vi "PrimaryInterfaceGetData.vi"(8 "PrimaryInterface":refnum<k24>, 11 "error in":errorcluster) -> (0 "Data":T1, 3 "error out":errorcluster)   [LabVIEW 2011, in "UnderAutomation.UniversalRobots.lvlib"]
uses:
  UnderAutomation.UniversalRobots.lvlib
  C:/Users/fg/Documents/UniversalRobots.vi/LabVIEW_2024/UnderAutomation.UniversalRobots/lib/UnderAutomation.UniversalRobots.dll
  LabVIEW_2024/UnderAutomation.UniversalRobots/lib/UnderAutomation.UniversalRobots.dll
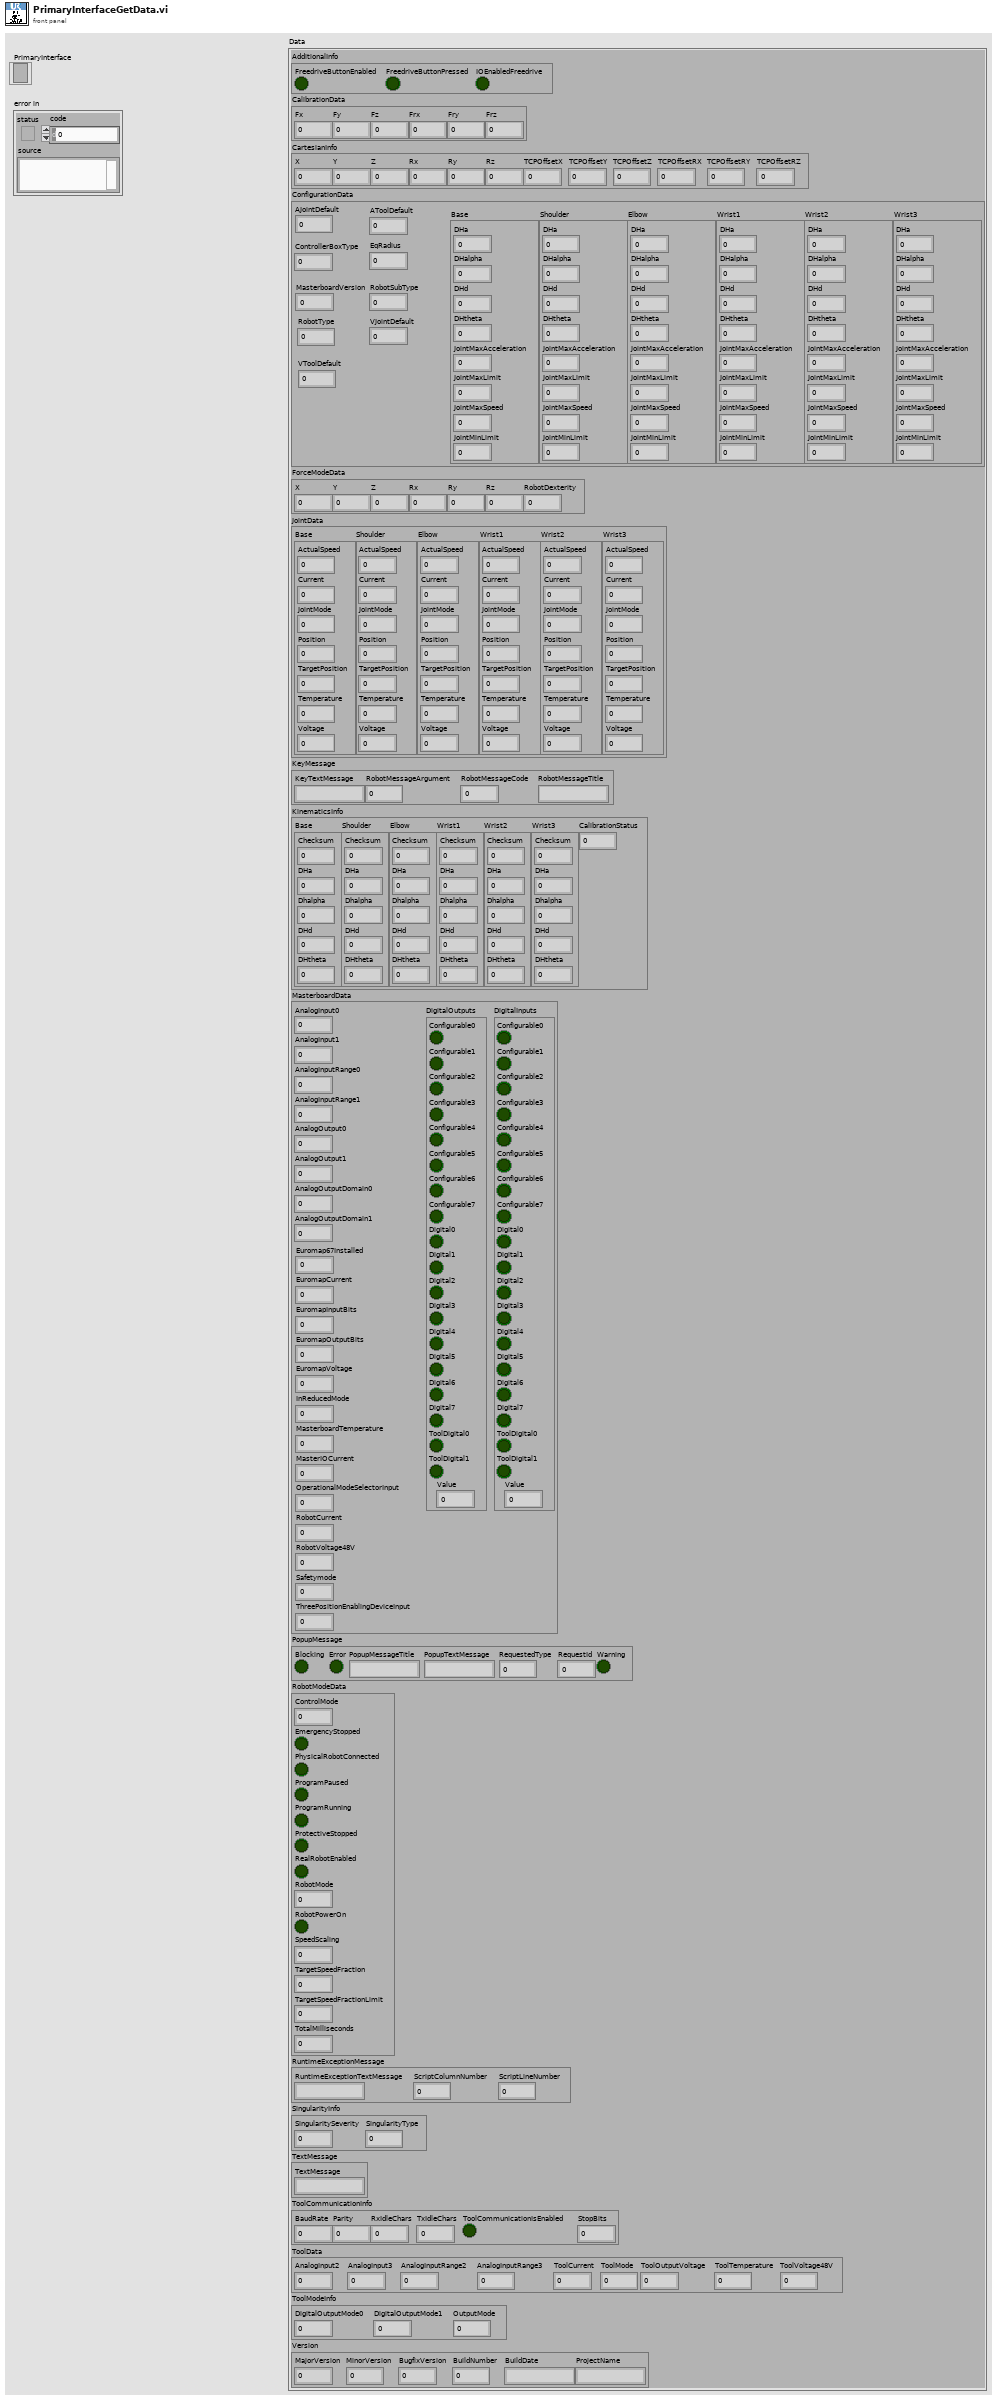
[diagram p1: front panel]
types:
  T1 = cluster{"AdditionalInfo":cluster{"FreedriveButtonEnabled":bool, "FreedriveButtonPressed":bool, "IOEnabledFreedrive":bool}, "CalibrationData":cluster{"Fx":dbl, "Fy":dbl, "Fz":dbl, "Frx":dbl, "Fry":dbl, "Frz":dbl}, "CartesianInfo":cluster{"X":dbl, "Y":dbl, "Z":dbl, "Rx":dbl, "Ry":dbl, "Rz":dbl, "TCPOffsetX":dbl, "TCPOffsetY":dbl, "TCPOffsetZ":dbl, "TCPOffsetRX":dbl, "TCPOffsetRY":dbl, "TCPOffsetRZ":dbl}, "ConfigurationData":cluster{"AJointDefault":dbl, "AToolDefault":dbl, "ControllerBoxType":i32, "EqRadius":dbl, "MasterboardVersion":i32, "RobotSubType":i32, "RobotType":i32, "VJointDefault":dbl, "VToolDefault":dbl, "Base":cluster{"DHa":dbl, "DHalpha":dbl, "DHd":dbl, "DHtheta":dbl, "JointMaxAcceleration":dbl, "JointMaxLimit":dbl, "JointMaxSpeed":dbl, "JointMinLimit":dbl}, "Shoulder":cluster{"DHa":dbl, "DHalpha":dbl, "DHd":dbl, "DHtheta":dbl, "JointMaxAcceleration":dbl, "JointMaxLimit":dbl, "JointMaxSpeed":dbl, "JointMinLimit":dbl}, "Elbow":cluster{"DHa":dbl, "DHalpha":dbl, "DHd":dbl, "DHtheta":dbl, "JointMaxAcceleration":dbl, "JointMaxLimit":dbl, "JointMaxSpeed":dbl, "JointMinLimit":dbl}, "Wrist1":cluster{"DHa":dbl, "DHalpha":dbl, "DHd":dbl, "DHtheta":dbl, "JointMaxAcceleration":dbl, "JointMaxLimit":dbl, "JointMaxSpeed":dbl, "JointMinLimit":dbl}, "Wrist2":cluster{"DHa":dbl, "DHalpha":dbl, "DHd":dbl, "DHtheta":dbl, "JointMaxAcceleration":dbl, "JointMaxLimit":dbl, "JointMaxSpeed":dbl, "JointMinLimit":dbl}, "Wrist3":cluster{"DHa":dbl, "DHalpha":dbl, "DHd":dbl, "DHtheta":dbl, "JointMaxAcceleration":dbl, "JointMaxLimit":dbl, "JointMaxSpeed":dbl, "JointMinLimit":dbl}}, "ForceModeData":cluster{"X":dbl, "Y":dbl, "Z":dbl, "Rx":dbl, "Ry":dbl, "Rz":dbl, "RobotDexterity":dbl}, "JointData":cluster{"Base":cluster{"ActualSpeed":dbl, "Current":sgl, "JointMode":u8, "Position":dbl, "TargetPosition":dbl, "Temperature":sgl, "Voltage":sgl}, "Shoulder":cluster{"ActualSpeed":dbl, "Current":sgl, "JointMode":u8, "Position":dbl, "TargetPosition":dbl, "Temperature":sgl, "Voltage":sgl}, "Elbow":cluster{"ActualSpeed":dbl, "Current":sgl, "JointMode":u8, "Position":dbl, "TargetPosition":dbl, "Temperature":sgl, "Voltage":sgl}, "Wrist1":cluster{"ActualSpeed":dbl, "Current":sgl, "JointMode":u8, "Position":dbl, "TargetPosition":dbl, "Temperature":sgl, "Voltage":sgl}, "Wrist2":cluster{"ActualSpeed":dbl, "Current":sgl, "JointMode":u8, "Position":dbl, "TargetPosition":dbl, "Temperature":sgl, "Voltage":sgl}, "Wrist3":cluster{"ActualSpeed":dbl, "Current":sgl, "JointMode":u8, "Position":dbl, "TargetPosition":dbl, "Temperature":sgl, "Voltage":sgl}}, "KeyMessage":cluster{"KeyTextMessage":string, "RobotMessageArgument":i32, "RobotMessageCode":i32, "RobotMessageTitle":string}, "KinematicsInfo":cluster{"Base":cluster{"Checksum":i32, "DHa":dbl, "Dhalpha":dbl, "DHd":dbl, "DHtheta":dbl}, "Shoulder":cluster{"Checksum":i32, "DHa":dbl, "Dhalpha":dbl, "DHd":dbl, "DHtheta":dbl}, "Elbow":cluster{"Checksum":i32, "DHa":dbl, "Dhalpha":dbl, "DHd":dbl, "DHtheta":dbl}, "Wrist1":cluster{"Checksum":i32, "DHa":dbl, "Dhalpha":dbl, "DHd":dbl, "DHtheta":dbl}, "Wrist2":cluster{"Checksum":i32, "DHa":dbl, "Dhalpha":dbl, "DHd":dbl, "DHtheta":dbl}, "Wrist3":cluster{"Checksum":i32, "DHa":dbl, "Dhalpha":dbl, "DHd":dbl, "DHtheta":dbl}, "CalibrationStatus":i32}, "MasterboardData":cluster{"AnalogInput0":dbl, "AnalogInput1":dbl, "AnalogInputRange0":i32, "AnalogInputRange1":i32, "AnalogOutput0":dbl, "AnalogOutput1":dbl, "AnalogOutputDomain0":i32, "AnalogOutputDomain1":i32, "DigitalInputs":cluster{"Configurable0":bool, "Configurable1":bool, "Configurable2":bool, "Configurable3":bool, "Configurable4":bool, "Configurable5":bool, "Configurable6":bool, "Configurable7":bool, "Digital0":bool, "Digital1":bool, "Digital2":bool, "Digital3":bool, "Digital4":bool, "Digital5":bool, "Digital6":bool, "Digital7":bool, "ToolDigital0":bool, "ToolDigital1":bool, "Value":i32}, "DigitalOutputs":cluster{"Configurable0":bool, "Configurable1":bool, "Configurable2":bool, "Configurable3":bool, "Configurable4":bool, "Configurable5":bool, "Configurable6":bool, "Configurable7":bool, "Digital0":bool, "Digital1":bool, "Digital2":bool, "Digital3":bool, "Digital4":bool, "Digital5":bool, "Digital6":bool, "Digital7":bool, "ToolDigital0":bool, "ToolDigital1":bool, "Value":i32}, "Euromap67Installed":i8, "EuromapCurrent":sgl, "EuromapInputBits":i32, "EuromapOutputBits":i32, "EuromapVoltage":sgl, "InReducedMode":u8, "MasterboardTemperature":sgl, "MasterIOCurrent":sgl, "OperationalModeSelectorInput":u8, "RobotCurrent":sgl, "RobotVoltage48V":sgl, "Safetymode":u8, "ThreePositionEnablingDeviceInput":u8}, "PopupMessage":cluster{"Blocking":bool, "Error":bool, "PopupMessageTitle":string, "PopupTextMessage":string, "RequestedType":i32, "RequestId":u32, "Warning":bool}, "RobotModeData":cluster{"ControlMode":i32, "EmergencyStopped":bool, "PhysicalRobotConnected":bool, "ProgramPaused":bool, "ProgramRunning":bool, "ProtectiveStopped":bool, "RealRobotEnabled":bool, "RobotMode":i32, "RobotPowerOn":bool, "SpeedScaling":dbl, "TargetSpeedFraction":dbl, "TargetSpeedFractionLimit":dbl, "TotalMilliseconds":dbl}, "RuntimeExceptionMessage":cluster{"RuntimeExceptionTextMessage":string, "ScriptColumnNumber":i32, "ScriptLineNumber":i32}, "SingularityInfo":cluster{"SingularitySeverity":u8, "SingularityType":u8}, "TextMessage":cluster{"TextMessage":string}, "ToolCommunicationInfo":cluster{"BaudRate":i32, "Parity":i32, "RxIdleChars":sgl, "TxIdleChars":sgl, "ToolCommunicationIsEnabled":bool, "StopBits":i32}, "ToolData":cluster{"AnalogInput2":dbl, "AnalogInput3":dbl, "AnalogInputRange2":i32, "AnalogInputRange3":i32, "ToolCurrent":sgl, "ToolMode":u8, "ToolOutputVoltage":i8, "ToolTemperature":sgl, "ToolVoltage48V":sgl}, "ToolModeInfo":cluster{"DigitalOutputMode0":i32, "DigitalOutputMode1":i32, "OutputMode":i32}, "Version":cluster{"MajorVersion":u8, "MinorVersion":u8, "BugfixVersion":i32, "BuildNumber":i32, "BuildDate":string, "ProjectName":string}}
  T2 = cluster{"X":dbl, "Y":dbl, "Z":dbl, "Rx":dbl, "Ry":dbl, "Rz":dbl, "TCPOffsetX":dbl, "TCPOffsetY":dbl, "TCPOffsetZ":dbl, "TCPOffsetRX":dbl, "TCPOffsetRY":dbl, "TCPOffsetRZ":dbl}
  T3 = cluster{"Blocking":bool, "Error":bool, "PopupMessageTitle":string, "PopupTextMessage":string, "RequestedType":i32, "RequestId":u32, "Warning":bool}
  T4 = cluster{"AnalogInput2":dbl, "AnalogInput3":dbl, "AnalogInputRange2":i32, "AnalogInputRange3":i32, "ToolCurrent":sgl, "ToolMode":u8, "ToolOutputVoltage":i8, "ToolTemperature":sgl, "ToolVoltage48V":sgl}
  T5 = cluster{"MajorVersion":u8, "MinorVersion":u8, "BugfixVersion":i32, "BuildNumber":i32, "BuildDate":string, "ProjectName":string}
  T6 = cluster{"X":dbl, "Y":dbl, "Z":dbl, "Rx":dbl, "Ry":dbl, "Rz":dbl, "RobotDexterity":dbl}
  T7 = cluster{"Fx":dbl, "Fy":dbl, "Fz":dbl, "Frx":dbl, "Fry":dbl, "Frz":dbl}
  T8 = cluster{"KeyTextMessage":string, "RobotMessageArgument":i32, "RobotMessageCode":i32, "RobotMessageTitle":string}
  T9 = cluster{"BaudRate":i32, "Parity":i32, "RxIdleChars":sgl, "TxIdleChars":sgl, "ToolCommunicationIsEnabled":bool, "StopBits":i32}
  T10 = cluster{"DHa":dbl, "DHalpha":dbl, "DHd":dbl, "DHtheta":dbl, "JointMaxAcceleration":dbl, "JointMaxLimit":dbl, "JointMaxSpeed":dbl, "JointMinLimit":dbl}
  T11 = cluster{"ActualSpeed":dbl, "Current":sgl, "JointMode":u8, "Position":dbl, "TargetPosition":dbl, "Temperature":sgl, "Voltage":sgl}
  T12 = cluster{"Checksum":i32, "DHa":dbl, "Dhalpha":dbl, "DHd":dbl, "DHtheta":dbl}
  T13 = cluster{"Configurable0":bool, "Configurable1":bool, "Configurable2":bool, "Configurable3":bool, "Configurable4":bool, "Configurable5":bool, "Configurable6":bool, "Configurable7":bool, "Digital0":bool, "Digital1":bool, "Digital2":bool, "Digital3":bool, "Digital4":bool, "Digital5":bool, "Digital6":bool, "Digital7":bool, "ToolDigital0":bool, "ToolDigital1":bool, "Value":i32}
  T14 = cluster{"ControlMode":i32, "EmergencyStopped":bool, "PhysicalRobotConnected":bool, "ProgramPaused":bool, "ProgramRunning":bool, "ProtectiveStopped":bool, "RealRobotEnabled":bool, "RobotMode":i32, "RobotPowerOn":bool, "SpeedScaling":dbl, "TargetSpeedFraction":dbl, "TargetSpeedFractionLimit":dbl, "TotalMilliseconds":dbl}
  T15 = cluster{"FreedriveButtonEnabled":bool, "FreedriveButtonPressed":bool, "IOEnabledFreedrive":bool}
  T16 = cluster{"AJointDefault":dbl, "AToolDefault":dbl, "ControllerBoxType":i32, "EqRadius":dbl, "MasterboardVersion":i32, "RobotSubType":i32, "RobotType":i32, "VJointDefault":dbl, "VToolDefault":dbl, cluster{"DHa":dbl, "DHalpha":dbl, "DHd":dbl, "DHtheta":dbl, "JointMaxAcceleration":dbl, "JointMaxLimit":dbl, "JointMaxSpeed":dbl, "JointMinLimit":dbl}, cluster{"DHa":dbl, "DHalpha":dbl, "DHd":dbl, "DHtheta":dbl, "JointMaxAcceleration":dbl, "JointMaxLimit":dbl, "JointMaxSpeed":dbl, "JointMinLimit":dbl}, cluster{"DHa":dbl, "DHalpha":dbl, "DHd":dbl, "DHtheta":dbl, "JointMaxAcceleration":dbl, "JointMaxLimit":dbl, "JointMaxSpeed":dbl, "JointMinLimit":dbl}, cluster{"DHa":dbl, "DHalpha":dbl, "DHd":dbl, "DHtheta":dbl, "JointMaxAcceleration":dbl, "JointMaxLimit":dbl, "JointMaxSpeed":dbl, "JointMinLimit":dbl}, cluster{"DHa":dbl, "DHalpha":dbl, "DHd":dbl, "DHtheta":dbl, "JointMaxAcceleration":dbl, "JointMaxLimit":dbl, "JointMaxSpeed":dbl, "JointMinLimit":dbl}, cluster{"DHa":dbl, "DHalpha":dbl, "DHd":dbl, "DHtheta":dbl, "JointMaxAcceleration":dbl, "JointMaxLimit":dbl, "JointMaxSpeed":dbl, "JointMinLimit":dbl}}
  T17 = cluster{cluster{"ActualSpeed":dbl, "Current":sgl, "JointMode":u8, "Position":dbl, "TargetPosition":dbl, "Temperature":sgl, "Voltage":sgl}, cluster{"ActualSpeed":dbl, "Current":sgl, "JointMode":u8, "Position":dbl, "TargetPosition":dbl, "Temperature":sgl, "Voltage":sgl}, cluster{"ActualSpeed":dbl, "Current":sgl, "JointMode":u8, "Position":dbl, "TargetPosition":dbl, "Temperature":sgl, "Voltage":sgl}, cluster{"ActualSpeed":dbl, "Current":sgl, "JointMode":u8, "Position":dbl, "TargetPosition":dbl, "Temperature":sgl, "Voltage":sgl}, cluster{"ActualSpeed":dbl, "Current":sgl, "JointMode":u8, "Position":dbl, "TargetPosition":dbl, "Temperature":sgl, "Voltage":sgl}, cluster{"ActualSpeed":dbl, "Current":sgl, "JointMode":u8, "Position":dbl, "TargetPosition":dbl, "Temperature":sgl, "Voltage":sgl}}
  T18 = cluster{cluster{"Checksum":i32, "DHa":dbl, "Dhalpha":dbl, "DHd":dbl, "DHtheta":dbl}, cluster{"Checksum":i32, "DHa":dbl, "Dhalpha":dbl, "DHd":dbl, "DHtheta":dbl}, cluster{"Checksum":i32, "DHa":dbl, "Dhalpha":dbl, "DHd":dbl, "DHtheta":dbl}, cluster{"Checksum":i32, "DHa":dbl, "Dhalpha":dbl, "DHd":dbl, "DHtheta":dbl}, cluster{"Checksum":i32, "DHa":dbl, "Dhalpha":dbl, "DHd":dbl, "DHtheta":dbl}, cluster{"Checksum":i32, "DHa":dbl, "Dhalpha":dbl, "DHd":dbl, "DHtheta":dbl}, "CalibrationStatus":i32}
  T19 = cluster{"AnalogInput0":dbl, "AnalogInput1":dbl, "AnalogInputRange0":i32, "AnalogInputRange1":i32, "AnalogOutput0":dbl, "AnalogOutput1":dbl, "AnalogOutputDomain0":i32, "AnalogOutputDomain1":i32, cluster{"Configurable0":bool, "Configurable1":bool, "Configurable2":bool, "Configurable3":bool, "Configurable4":bool, "Configurable5":bool, "Configurable6":bool, "Configurable7":bool, "Digital0":bool, "Digital1":bool, "Digital2":bool, "Digital3":bool, "Digital4":bool, "Digital5":bool, "Digital6":bool, "Digital7":bool, "ToolDigital0":bool, "ToolDigital1":bool, "Value":i32}, cluster{"Configurable0":bool, "Configurable1":bool, "Configurable2":bool, "Configurable3":bool, "Configurable4":bool, "Configurable5":bool, "Configurable6":bool, "Configurable7":bool, "Digital0":bool, "Digital1":bool, "Digital2":bool, "Digital3":bool, "Digital4":bool, "Digital5":bool, "Digital6":bool, "Digital7":bool, "ToolDigital0":bool, "ToolDigital1":bool, "Value":i32}, "Euromap67Installed":i8, "EuromapCurrent":sgl, "EuromapInputBits":i32, "EuromapOutputBits":i32, "EuromapVoltage":sgl, "InReducedMode":u8, "MasterboardTemperature":sgl, "MasterIOCurrent":sgl, "OperationalModeSelectorInput":u8, "RobotCurrent":sgl, "RobotVoltage48V":sgl, "Safetymode":u8, "ThreePositionEnablingDeviceInput":u8}
  T20 = cluster{"RuntimeExceptionTextMessage":string, "ScriptColumnNumber":i32, "ScriptLineNumber":i32}
  T21 = cluster{"SingularitySeverity":u8, "SingularityType":u8}
  T22 = cluster{"DigitalOutputMode0":i32, "DigitalOutputMode1":i32, "OutputMode":i32}
  T23 = cluster{cluster{"FreedriveButtonEnabled":bool, "FreedriveButtonPressed":bool, "IOEnabledFreedrive":bool}, cluster{"Fx":dbl, "Fy":dbl, "Fz":dbl, "Frx":dbl, "Fry":dbl, "Frz":dbl}, cluster{"X":dbl, "Y":dbl, "Z":dbl, "Rx":dbl, "Ry":dbl, "Rz":dbl, "TCPOffsetX":dbl, "TCPOffsetY":dbl, "TCPOffsetZ":dbl, "TCPOffsetRX":dbl, "TCPOffsetRY":dbl, "TCPOffsetRZ":dbl}, cluster{"AJointDefault":dbl, "AToolDefault":dbl, "ControllerBoxType":i32, "EqRadius":dbl, "MasterboardVersion":i32, "RobotSubType":i32, "RobotType":i32, "VJointDefault":dbl, "VToolDefault":dbl, cluster{"DHa":dbl, "DHalpha":dbl, "DHd":dbl, "DHtheta":dbl, "JointMaxAcceleration":dbl, "JointMaxLimit":dbl, "JointMaxSpeed":dbl, "JointMinLimit":dbl}, cluster{"DHa":dbl, "DHalpha":dbl, "DHd":dbl, "DHtheta":dbl, "JointMaxAcceleration":dbl, "JointMaxLimit":dbl, "JointMaxSpeed":dbl, "JointMinLimit":dbl}, cluster{"DHa":dbl, "DHalpha":dbl, "DHd":dbl, "DHtheta":dbl, "JointMaxAcceleration":dbl, "JointMaxLimit":dbl, "JointMaxSpeed":dbl, "JointMinLimit":dbl}, cluster{"DHa":dbl, "DHalpha":dbl, "DHd":dbl, "DHtheta":dbl, "JointMaxAcceleration":dbl, "JointMaxLimit":dbl, "JointMaxSpeed":dbl, "JointMinLimit":dbl}, cluster{"DHa":dbl, "DHalpha":dbl, "DHd":dbl, "DHtheta":dbl, "JointMaxAcceleration":dbl, "JointMaxLimit":dbl, "JointMaxSpeed":dbl, "JointMinLimit":dbl}, cluster{"DHa":dbl, "DHalpha":dbl, "DHd":dbl, "DHtheta":dbl, "JointMaxAcceleration":dbl, "JointMaxLimit":dbl, "JointMaxSpeed":dbl, "JointMinLimit":dbl}}, cluster{"X":dbl, "Y":dbl, "Z":dbl, "Rx":dbl, "Ry":dbl, "Rz":dbl, "RobotDexterity":dbl}, cluster{cluster{"ActualSpeed":dbl, "Current":sgl, "JointMode":u8, "Position":dbl, "TargetPosition":dbl, "Temperature":sgl, "Voltage":sgl}, cluster{"ActualSpeed":dbl, "Current":sgl, "JointMode":u8, "Position":dbl, "TargetPosition":dbl, "Temperature":sgl, "Voltage":sgl}, cluster{"ActualSpeed":dbl, "Current":sgl, "JointMode":u8, "Position":dbl, "TargetPosition":dbl, "Temperature":sgl, "Voltage":sgl}, cluster{"ActualSpeed":dbl, "Current":sgl, "JointMode":u8, "Position":dbl, "TargetPosition":dbl, "Temperature":sgl, "Voltage":sgl}, cluster{"ActualSpeed":dbl, "Current":sgl, "JointMode":u8, "Position":dbl, "TargetPosition":dbl, "Temperature":sgl, "Voltage":sgl}, cluster{"ActualSpeed":dbl, "Current":sgl, "JointMode":u8, "Position":dbl, "TargetPosition":dbl, "Temperature":sgl, "Voltage":sgl}}, cluster{"KeyTextMessage":string, "RobotMessageArgument":i32, "RobotMessageCode":i32, "RobotMessageTitle":string}, cluster{cluster{"Checksum":i32, "DHa":dbl, "Dhalpha":dbl, "DHd":dbl, "DHtheta":dbl}, cluster{"Checksum":i32, "DHa":dbl, "Dhalpha":dbl, "DHd":dbl, "DHtheta":dbl}, cluster{"Checksum":i32, "DHa":dbl, "Dhalpha":dbl, "DHd":dbl, "DHtheta":dbl}, cluster{"Checksum":i32, "DHa":dbl, "Dhalpha":dbl, "DHd":dbl, "DHtheta":dbl}, cluster{"Checksum":i32, "DHa":dbl, "Dhalpha":dbl, "DHd":dbl, "DHtheta":dbl}, cluster{"Checksum":i32, "DHa":dbl, "Dhalpha":dbl, "DHd":dbl, "DHtheta":dbl}, "CalibrationStatus":i32}, cluster{"AnalogInput0":dbl, "AnalogInput1":dbl, "AnalogInputRange0":i32, "AnalogInputRange1":i32, "AnalogOutput0":dbl, "AnalogOutput1":dbl, "AnalogOutputDomain0":i32, "AnalogOutputDomain1":i32, cluster{"Configurable0":bool, "Configurable1":bool, "Configurable2":bool, "Configurable3":bool, "Configurable4":bool, "Configurable5":bool, "Configurable6":bool, "Configurable7":bool, "Digital0":bool, "Digital1":bool, "Digital2":bool, "Digital3":bool, "Digital4":bool, "Digital5":bool, "Digital6":bool, "Digital7":bool, "ToolDigital0":bool, "ToolDigital1":bool, "Value":i32}, cluster{"Configurable0":bool, "Configurable1":bool, "Configurable2":bool, "Configurable3":bool, "Configurable4":bool, "Configurable5":bool, "Configurable6":bool, "Configurable7":bool, "Digital0":bool, "Digital1":bool, "Digital2":bool, "Digital3":bool, "Digital4":bool, "Digital5":bool, "Digital6":bool, "Digital7":bool, "ToolDigital0":bool, "ToolDigital1":bool, "Value":i32}, "Euromap67Installed":i8, "EuromapCurrent":sgl, "EuromapInputBits":i32, "EuromapOutputBits":i32, "EuromapVoltage":sgl, "InReducedMode":u8, "MasterboardTemperature":sgl, "MasterIOCurrent":sgl, "OperationalModeSelectorInput":u8, "RobotCurrent":sgl, "RobotVoltage48V":sgl, "Safetymode":u8, "ThreePositionEnablingDeviceInput":u8}, cluster{"Blocking":bool, "Error":bool, "PopupMessageTitle":string, "PopupTextMessage":string, "RequestedType":i32, "RequestId":u32, "Warning":bool}, cluster{"ControlMode":i32, "EmergencyStopped":bool, "PhysicalRobotConnected":bool, "ProgramPaused":bool, "ProgramRunning":bool, "ProtectiveStopped":bool, "RealRobotEnabled":bool, "RobotMode":i32, "RobotPowerOn":bool, "SpeedScaling":dbl, "TargetSpeedFraction":dbl, "TargetSpeedFractionLimit":dbl, "TotalMilliseconds":dbl}, cluster{"RuntimeExceptionTextMessage":string, "ScriptColumnNumber":i32, "ScriptLineNumber":i32}, cluster{"SingularitySeverity":u8, "SingularityType":u8}, cluster{"TextMessage":string}, cluster{"BaudRate":i32, "Parity":i32, "RxIdleChars":sgl, "TxIdleChars":sgl, "ToolCommunicationIsEnabled":bool, "StopBits":i32}, cluster{"AnalogInput2":dbl, "AnalogInput3":dbl, "AnalogInputRange2":i32, "AnalogInputRange3":i32, "ToolCurrent":sgl, "ToolMode":u8, "ToolOutputVoltage":i8, "ToolTemperature":sgl, "ToolVoltage48V":sgl}, cluster{"DigitalOutputMode0":i32, "DigitalOutputMode1":i32, "OutputMode":i32}, cluster{"MajorVersion":u8, "MinorVersion":u8, "BugfixVersion":i32, "BuildNumber":i32, "BuildDate":string, "ProjectName":string}}
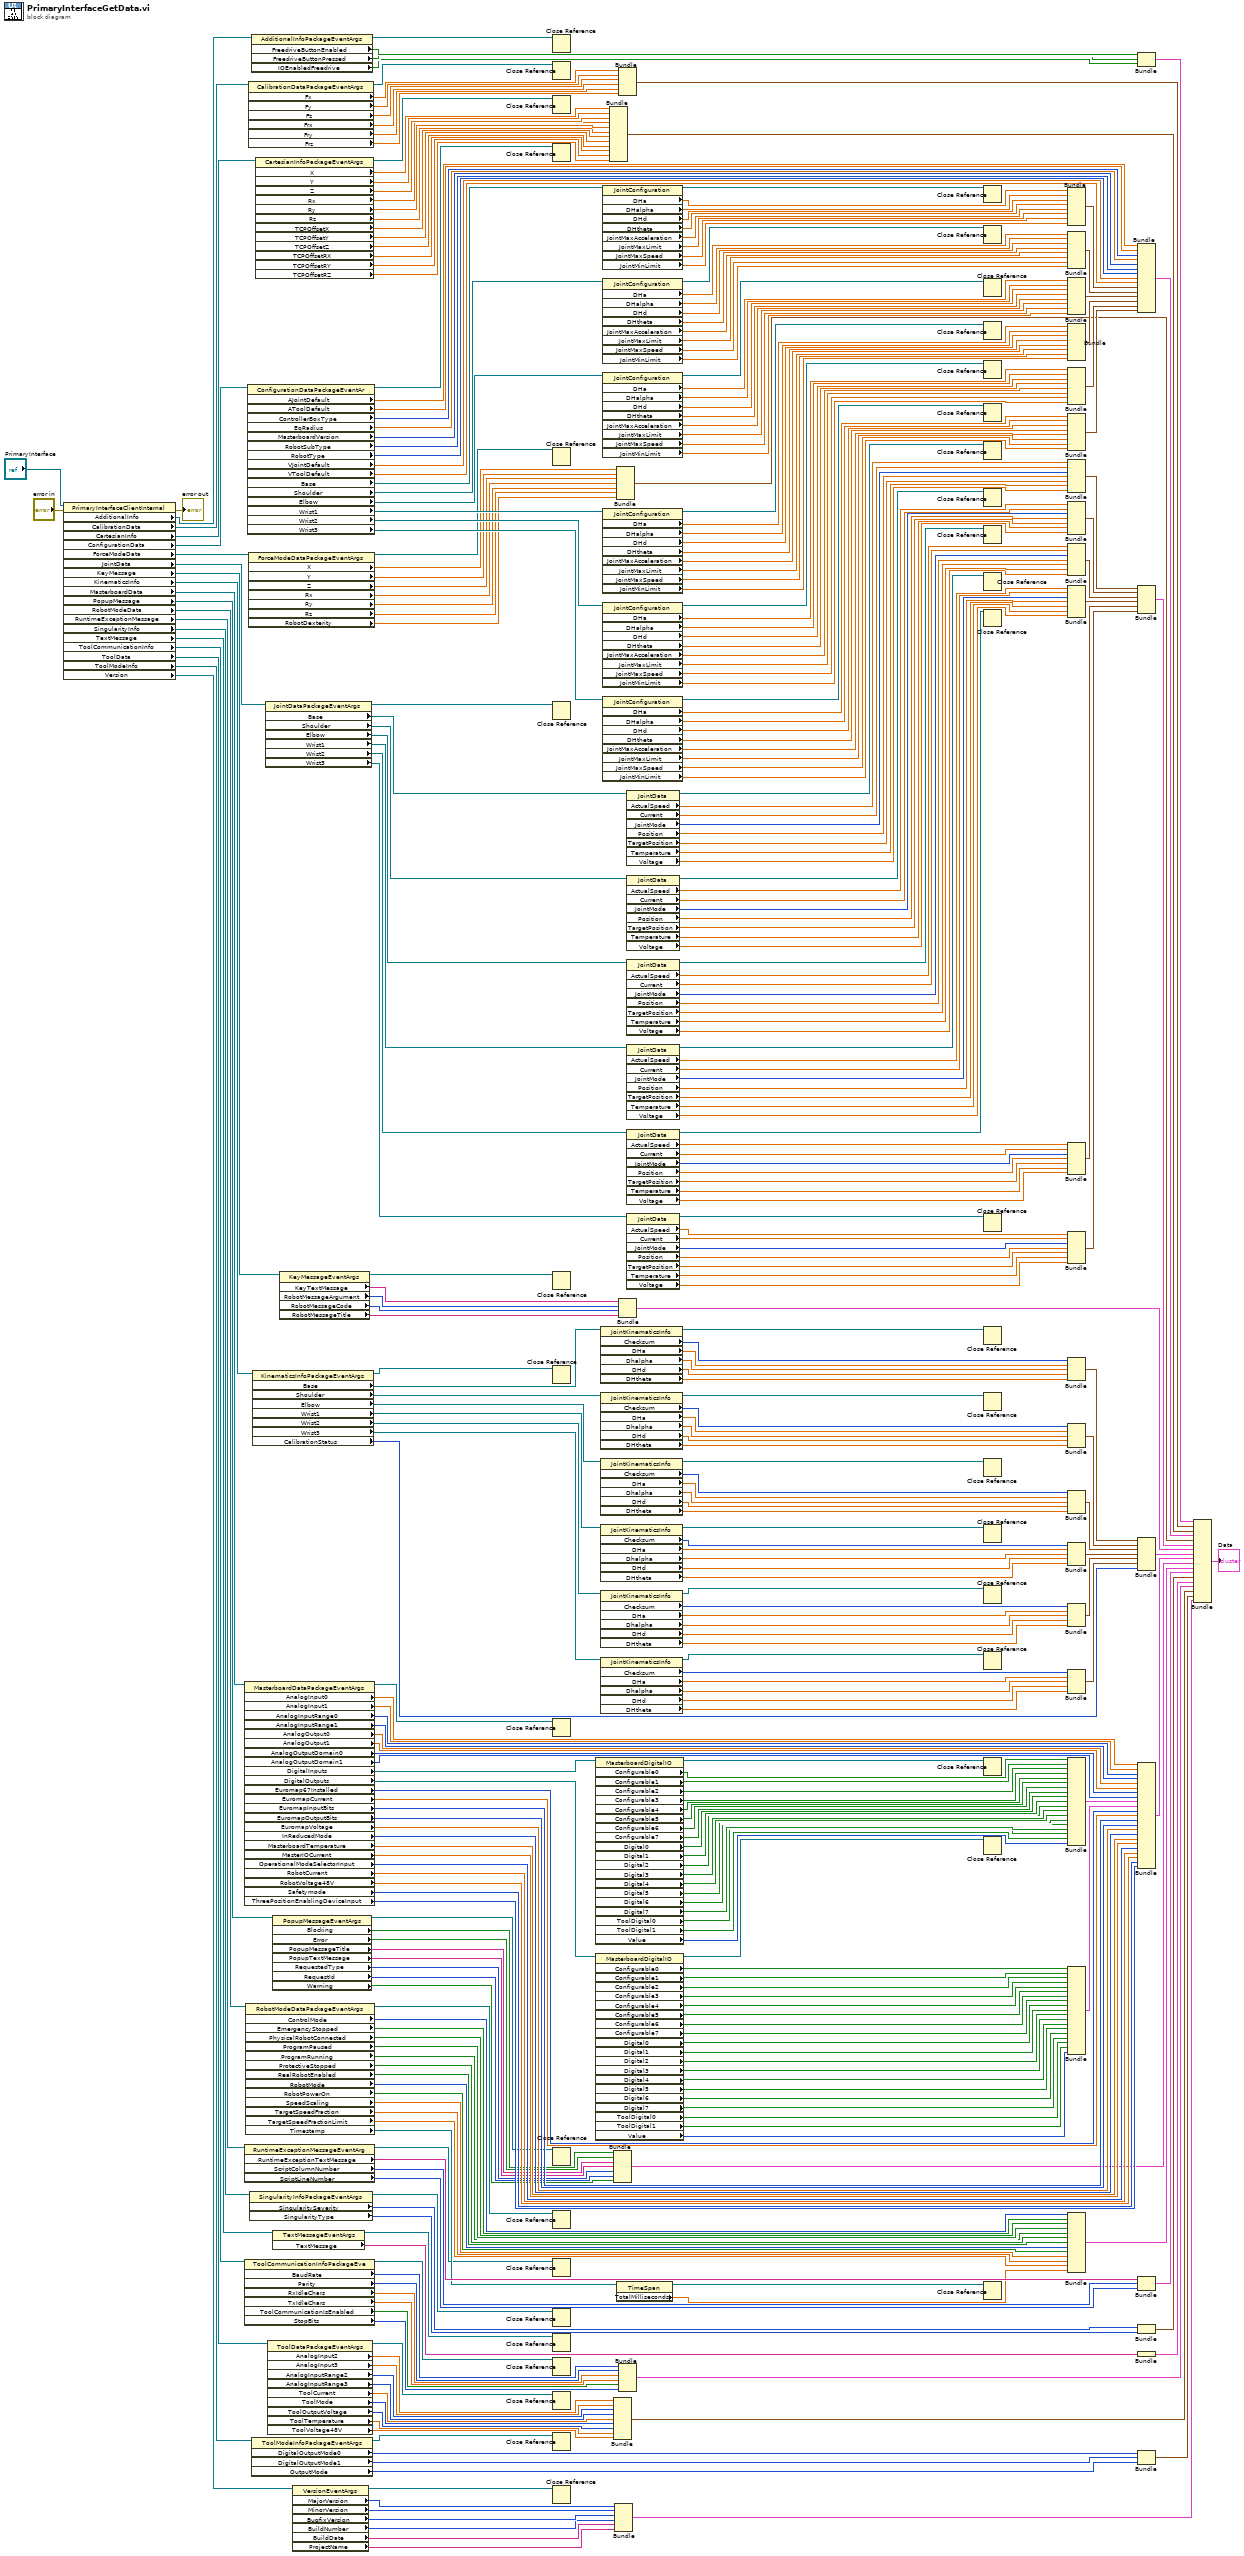
[diagram p0: block diagram]
diagram:
  n1 = property class="PrimaryInterfaceClientInternal"(reference="PrimaryInterface", error in="error in") -> (error out=→"error out":errorcluster, "AdditionalInfo"=w246:refnum<k24>, "CalibrationData"=w243:refnum<k24>, "CartesianInfo"=w244:refnum<k24>, "ConfigurationData"=w248:refnum<k24>, "ForceModeData"=w245:refnum<k24>, "JointData"=w236:refnum<k24>, "KeyMessage"=w181:refnum<k24>, "KinematicsInfo"=w249:refnum<k24>, "MasterboardData"=w175:refnum<k24>, "PopupMessage"=w111:refnum<k24>, "RobotModeData"=w103:refnum<k24>, "RuntimeExceptionMessage"=w87:refnum<k24>, "SingularityInfo"=w83:refnum<k24>, "TextMessage"=w79:refnum<k24>, "ToolCommunicationInfo"=w76:refnum<k24>, "ToolData"=w68:refnum<k24>, "ToolModeInfo"=w58:refnum<k24>, "Version"=w247:refnum<k24>)  [unwired: 1 out]
  n2 = property class="MasterboardDataPackageEventArgs"(reference=w175) -> (reference out=w14:refnum<k24>, "AnalogInput0"=w135:dbl, "AnalogInput1"=w134:dbl, "AnalogInputRange0"=w133:i32, "AnalogInputRange1"=w132:i32, "AnalogOutput0"=w131:dbl, "AnalogOutput1"=w130:dbl, "AnalogOutputDomain0"=w129:i32, "AnalogOutputDomain1"=w128:i32, "DigitalInputs"=w176:refnum<k24>, "DigitalOutputs"=w136:refnum<k24>, "Euromap67Installed"=w125:i8, "EuromapCurrent"=w124:sgl, "EuromapInputBits"=w123:i32, "EuromapOutputBits"=w122:i32, "EuromapVoltage"=w121:sgl, "InReducedMode"=w120:u8, "MasterboardTemperature"=w119:sgl, "MasterIOCurrent"=w118:sgl, "OperationalModeSelectorInput"=w117:u8, "RobotCurrent"=w116:sgl, "RobotVoltage48V"=w115:sgl, "Safetymode"=w114:u8, "ThreePositionEnablingDeviceInput"=w113:u8)  [unwired: 1 in, 1 out]
  n3 = property class="RuntimeExceptionMessageEventArg"(reference=w87) -> (reference out=w9:refnum<k24>, "RuntimeExceptionTextMessage"=w90:string, "ScriptColumnNumber"=w89:i32, "ScriptLineNumber"=w88:i32)  [unwired: 1 in, 1 out]
  n4 = property class="ToolCommunicationInfoPackageEve"(reference=w76) -> (reference out=w5:refnum<k24>, "BaudRate"=w75:i32, "Parity"=w74:i32, "RxIdleChars"=w73:sgl, "TxIdleChars"=w72:sgl, "ToolCommunicationIsEnabled"=w71:bool, "StopBits"=w70:i32)  [unwired: 1 in, 1 out]
  n5 = property class="RobotModeDataPackageEventArgs"(reference=w103) -> (reference out=w10:refnum<k24>, "ControlMode"=w102:i32, "EmergencyStopped"=w101:bool, "PhysicalRobotConnected"=w100:bool, "ProgramPaused"=w99:bool, "ProgramRunning"=w98:bool, "ProtectiveStopped"=w97:bool, "RealRobotEnabled"=w96:bool, "RobotMode"=w95:i32, "RobotPowerOn"=w94:bool, "SpeedScaling"=w93:dbl, "TargetSpeedFraction"=w92:dbl, "TargetSpeedFractionLimit"=w91:dbl, "Timestamp"=w50:refnum<k24>)  [unwired: 1 in, 1 out]
  n6 = property class="ConfigurationDataPackageEventAr"(reference=w248) -> (reference out=w37:refnum<k24>, "AJointDefault"=w336:dbl, "AToolDefault"=w335:dbl, "ControllerBoxType"=w334:i32, "EqRadius"=w333:dbl, "MasterboardVersion"=w332:i32, "RobotSubType"=w331:i32, "RobotType"=w330:i32, "VJointDefault"=w329:dbl, "VToolDefault"=w328:dbl, "Base"=w390:refnum<k24>, "Shoulder"=w341:refnum<k24>, "Elbow"=w340:refnum<k24>, "Wrist1"=w339:refnum<k24>, "Wrist2"=w338:refnum<k24>, "Wrist3"=w337:refnum<k24>)  [unwired: 1 in, 1 out]
  n7 = property class="ForceModeDataPackageEventArgs"(reference=w245) -> (reference out=w30:refnum<k24>, "X"=w256:dbl, "Y"=w255:dbl, "Z"=w254:dbl, "Rx"=w253:dbl, "Ry"=w252:dbl, "Rz"=w251:dbl, "RobotDexterity"=w250:dbl)  [unwired: 1 in, 1 out]
  n8 = property class="CalibrationDataPackageEventArgs"(reference=w243) -> (reference out=w39:refnum<k24>, "Fx"=w242:dbl, "Fy"=w241:dbl, "Fz"=w240:dbl, "Frx"=w239:dbl, "Fry"=w238:dbl, "Frz"=w237:dbl)  [unwired: 1 in, 1 out]
  n9 = property class="SingularityInfoPackageEventArgs"(reference=w83) -> (reference out=w8:refnum<k24>, "SingularitySeverity"=w82:u8, "SingularityType"=w81:u8)  [unwired: 1 in, 1 out]
  n10 = property class="AdditionalInfoPackageEventArgs"(reference=w246) -> (reference out=w40:refnum<k24>, "FreedriveButtonEnabled"=w271:bool, "FreedriveButtonPressed"=w270:bool, "IOEnabledFreedrive"=w269:bool)  [unwired: 1 in, 1 out]
  n11 = property class="ToolModeInfoPackageEventArgs"(reference=w58) -> (reference out=w3:refnum<k24>, "DigitalOutputMode0"=w57:i32, "DigitalOutputMode1"=w56:i32, "OutputMode"=w55:i32)  [unwired: 1 in, 1 out]
  n12 = property class="KinematicsInfoPackageEventArgs"(reference=w249) -> (reference out=w15:refnum<k24>, "Base"=w321:refnum<k24>, "Shoulder"=w290:refnum<k24>, "Elbow"=w289:refnum<k24>, "Wrist1"=w288:refnum<k24>, "Wrist2"=w287:refnum<k24>, "Wrist3"=w286:refnum<k24>, "CalibrationStatus"=w279:i32)  [unwired: 1 in, 1 out]
  n13 = property class="CartesianInfoPackageEventArgs"(reference=w244) -> (reference out=w38:refnum<k24>, "X"=w268:dbl, "Y"=w267:dbl, "Z"=w266:dbl, "Rx"=w265:dbl, "Ry"=w264:dbl, "Rz"=w263:dbl, "TCPOffsetX"=w262:dbl, "TCPOffsetY"=w260:dbl, "TCPOffsetZ"=w261:dbl, "TCPOffsetRX"=w258:dbl, "TCPOffsetRY"=w259:dbl, "TCPOffsetRZ"=w257:dbl)  [unwired: 1 in, 1 out]
  n14 = property class="JointDataPackageEventArgs"(reference=w236) -> (reference out=w25:refnum<k24>, "Base"=w235:refnum<k24>, "Shoulder"=w192:refnum<k24>, "Elbow"=w191:refnum<k24>, "Wrist1"=w190:refnum<k24>, "Wrist2"=w189:refnum<k24>, "Wrist3"=w188:refnum<k24>)  [unwired: 1 in, 1 out]
  n15 = property class="ToolDataPackageEventArgs"(reference=w68) -> (reference out=w4:refnum<k24>, "AnalogInput2"=w67:dbl, "AnalogInput3"=w66:dbl, "AnalogInputRange2"=w65:i32, "AnalogInputRange3"=w64:i32, "ToolCurrent"=w63:sgl, "ToolMode"=w62:u8, "ToolOutputVoltage"=w61:i8, "ToolTemperature"=w60:sgl, "ToolVoltage48V"=w59:sgl)  [unwired: 1 in, 1 out]
  n16 = property class="PopupMessageEventArgs"(reference=w111) -> (reference out=w11:refnum<k24>, "Blocking"=w110:bool, "Error"=w109:bool, "PopupMessageTitle"=w108:string, "PopupTextMessage"=w107:string, "RequestedType"=w106:i32, "RequestId"=w105:u32, "Warning"=w104:bool)  [unwired: 1 in, 1 out]
  n17 = property class="TextMessageEventArgs"(reference=w79) -> (reference out=w7:refnum<k24>, "TextMessage"=w78:string)  [unwired: 1 in, 1 out]
  n18 = property class="KeyMessageEventArgs"(reference=w181) -> (reference out=w16:refnum<k24>, "KeyTextMessage"=w180:string, "RobotMessageArgument"=w179:i32, "RobotMessageCode"=w178:i32, "RobotMessageTitle"=w177:string)  [unwired: 1 in, 1 out]
  n19 = property class="VersionEventArgs"(reference=w247) -> (reference out=w2:refnum<k24>, "MajorVersion"=w278:u8, "MinorVersion"=w277:u8, "BugfixVersion"=w276:i32, "BuildNumber"=w275:i32, "BuildDate"=w274:string, "ProjectName"=w273:string)  [unwired: 1 in, 1 out]
  n20 = Close Reference(reference=w40) -> ()  [unwired: 1 in, 1 out]
  n21 = Close Reference(reference=w39) -> ()  [unwired: 1 in, 1 out]
  n22 = Close Reference(reference=w38) -> ()  [unwired: 1 in, 1 out]
  n23 = Close Reference(reference=w37) -> ()  [unwired: 1 in, 1 out]
  n24 = Close Reference(reference=w30) -> ()  [unwired: 1 in, 1 out]
  n25 = Close Reference(reference=w25) -> ()  [unwired: 1 in, 1 out]
  n26 = Close Reference(reference=w16) -> ()  [unwired: 1 in, 1 out]
  n27 = Close Reference(reference=w15) -> ()  [unwired: 1 in, 1 out]
  n28 = Close Reference(reference=w14) -> ()  [unwired: 1 in, 1 out]
  n29 = Close Reference(reference=w11) -> ()  [unwired: 1 in, 1 out]
  n30 = Close Reference(reference=w10) -> ()  [unwired: 1 in, 1 out]
  n31 = Close Reference(reference=w9) -> ()  [unwired: 1 in, 1 out]
  n32 = Close Reference(reference=w8) -> ()  [unwired: 1 in, 1 out]
  n33 = Close Reference(reference=w7) -> ()  [unwired: 1 in, 1 out]
  n34 = Close Reference(reference=w5) -> ()  [unwired: 1 in, 1 out]
  n35 = Close Reference(reference=w4) -> ()  [unwired: 1 in, 1 out]
  n36 = Close Reference(reference=w3) -> ()  [unwired: 1 in, 1 out]
  n37 = Close Reference(reference=w2) -> ()  [unwired: 1 in, 1 out]
  n38 = property class="MasterboardDigitalIO"(reference=w176) -> (reference out=w13:refnum<k24>, "Configurable0"=w174:bool, "Configurable1"=w173:bool, "Configurable2"=w172:bool, "Configurable3"=w171:bool, "Configurable4"=w170:bool, "Configurable5"=w169:bool, "Configurable6"=w168:bool, "Configurable7"=w167:bool, "Digital0"=w166:bool, "Digital1"=w165:bool, "Digital2"=w164:bool, "Digital3"=w163:bool, "Digital4"=w162:bool, "Digital5"=w161:bool, "Digital6"=w160:bool, "Digital7"=w159:bool, "ToolDigital0"=w158:bool, "ToolDigital1"=w157:bool, "Value"=w156:i32)  [unwired: 1 in, 1 out]
  n39 = property class="MasterboardDigitalIO"(reference=w136) -> (reference out=w12:refnum<k24>, "Configurable0"=w137:bool, "Configurable1"=w138:bool, "Configurable2"=w139:bool, "Configurable3"=w140:bool, "Configurable4"=w141:bool, "Configurable5"=w142:bool, "Configurable6"=w143:bool, "Configurable7"=w144:bool, "Digital0"=w145:bool, "Digital1"=w146:bool, "Digital2"=w147:bool, "Digital3"=w148:bool, "Digital4"=w149:bool, "Digital5"=w150:bool, "Digital6"=w151:bool, "Digital7"=w152:bool, "ToolDigital0"=w153:bool, "ToolDigital1"=w154:bool, "Value"=w155:i32)  [unwired: 1 in, 1 out]
  n40 = property class="JointKinematicsInfo"(reference=w321) -> (reference out=w22:refnum<k24>, "Checksum"=w320:i32, "DHa"=w319:dbl, "Dhalpha"=w318:dbl, "DHd"=w317:dbl, "DHtheta"=w316:dbl)  [unwired: 1 in, 1 out]
  n41 = property class="JointKinematicsInfo"(reference=w290) -> (reference out=w21:refnum<k24>, "Checksum"=w311:i32, "DHa"=w312:dbl, "Dhalpha"=w313:dbl, "DHd"=w314:dbl, "DHtheta"=w315:dbl)  [unwired: 1 in, 1 out]
  n42 = property class="JointKinematicsInfo"(reference=w289) -> (reference out=w20:refnum<k24>, "Checksum"=w310:i32, "DHa"=w309:dbl, "Dhalpha"=w308:dbl, "DHd"=w307:dbl, "DHtheta"=w306:dbl)  [unwired: 1 in, 1 out]
  n43 = property class="JointKinematicsInfo"(reference=w288) -> (reference out=w19:refnum<k24>, "Checksum"=w301:i32, "DHa"=w302:dbl, "Dhalpha"=w303:dbl, "DHd"=w304:dbl, "DHtheta"=w305:dbl)  [unwired: 1 in, 1 out]
  n44 = property class="JointKinematicsInfo"(reference=w287) -> (reference out=w18:refnum<k24>, "Checksum"=w300:i32, "DHa"=w299:dbl, "Dhalpha"=w298:dbl, "DHd"=w297:dbl, "DHtheta"=w296:dbl)  [unwired: 1 in, 1 out]
  n45 = property class="JointKinematicsInfo"(reference=w286) -> (reference out=w17:refnum<k24>, "Checksum"=w291:i32, "DHa"=w292:dbl, "Dhalpha"=w293:dbl, "DHd"=w294:dbl, "DHtheta"=w295:dbl)  [unwired: 1 in, 1 out]
  n46 = property class="JointConfiguration"(reference=w390) -> (reference out=w36:refnum<k24>, "DHa"=w389:dbl, "DHalpha"=w388:dbl, "DHd"=w387:dbl, "DHtheta"=w385:dbl, "JointMaxAcceleration"=w386:dbl, "JointMaxLimit"=w384:dbl, "JointMaxSpeed"=w383:dbl, "JointMinLimit"=w382:dbl)  [unwired: 1 in, 1 out]
  n47 = property class="JointConfiguration"(reference=w341) -> (reference out=w35:refnum<k24>, "DHa"=w342:dbl, "DHalpha"=w343:dbl, "DHd"=w344:dbl, "DHtheta"=w346:dbl, "JointMaxAcceleration"=w345:dbl, "JointMaxLimit"=w347:dbl, "JointMaxSpeed"=w348:dbl, "JointMinLimit"=w349:dbl)  [unwired: 1 in, 1 out]
  n48 = property class="JointConfiguration"(reference=w340) -> (reference out=w34:refnum<k24>, "DHa"=w357:dbl, "DHalpha"=w356:dbl, "DHd"=w355:dbl, "DHtheta"=w353:dbl, "JointMaxAcceleration"=w354:dbl, "JointMaxLimit"=w352:dbl, "JointMaxSpeed"=w351:dbl, "JointMinLimit"=w350:dbl)  [unwired: 1 in, 1 out]
  n49 = property class="JointConfiguration"(reference=w339) -> (reference out=w33:refnum<k24>, "DHa"=w374:dbl, "DHalpha"=w375:dbl, "DHd"=w376:dbl, "DHtheta"=w378:dbl, "JointMaxAcceleration"=w377:dbl, "JointMaxLimit"=w379:dbl, "JointMaxSpeed"=w380:dbl, "JointMinLimit"=w381:dbl)  [unwired: 1 in, 1 out]
  n50 = property class="JointConfiguration"(reference=w338) -> (reference out=w32:refnum<k24>, "DHa"=w373:dbl, "DHalpha"=w372:dbl, "DHd"=w371:dbl, "DHtheta"=w369:dbl, "JointMaxAcceleration"=w370:dbl, "JointMaxLimit"=w368:dbl, "JointMaxSpeed"=w367:dbl, "JointMinLimit"=w366:dbl)  [unwired: 1 in, 1 out]
  n51 = property class="JointConfiguration"(reference=w337) -> (reference out=w31:refnum<k24>, "DHa"=w358:dbl, "DHalpha"=w359:dbl, "DHd"=w360:dbl, "DHtheta"=w362:dbl, "JointMaxAcceleration"=w361:dbl, "JointMaxLimit"=w363:dbl, "JointMaxSpeed"=w364:dbl, "JointMinLimit"=w365:dbl)  [unwired: 1 in, 1 out]
  n52 = Bundle("X"=w268, "Y"=w267, "Z"=w266, "Rx"=w265, "Ry"=w264, "Rz"=w263, "TCPOffsetX"=w262, "TCPOffsetY"=w260, "TCPOffsetZ"=w261, "TCPOffsetRX"=w258, "TCPOffsetRY"=w259, "TCPOffsetRZ"=w257) -> (w45:T2)  [unwired: 1 in]
  n53 = Bundle("Blocking"=w110, "Error"=w109, "PopupMessageTitle"=w108, "PopupTextMessage"=w107, "RequestedType"=w106, "RequestId"=w105, "Warning"=w104) -> (w86:T3)  [unwired: 1 in]
  n54 = Bundle("AnalogInput2"=w67, "AnalogInput3"=w66, "AnalogInputRange2"=w65, "AnalogInputRange3"=w64, "ToolCurrent"=w63, "ToolMode"=w62, "ToolOutputVoltage"=w61, "ToolTemperature"=w60, "ToolVoltage48V"=w59) -> (w54:T4)  [unwired: 1 in]
  n55 = Bundle("MajorVersion"=w278, "MinorVersion"=w277, "BugfixVersion"=w276, "BuildNumber"=w275, "BuildDate"=w274, "ProjectName"=w273) -> (w52:T5)  [unwired: 1 in]
  n56 = Bundle("X"=w256, "Y"=w255, "Z"=w254, "Rx"=w253, "Ry"=w252, "Rz"=w251, "RobotDexterity"=w250) -> (w47:T6)  [unwired: 1 in]
  n57 = property class="TimeSpan"(reference=w50) -> (reference out=w6:refnum<k24>, "TotalMilliseconds"=w51:dbl)  [unwired: 1 in, 1 out]
  n58 = Bundle("Fx"=w242, "Fy"=w241, "Fz"=w240, "Frx"=w239, "Fry"=w238, "Frz"=w237) -> (w44:T7)  [unwired: 1 in]
  n59 = Bundle("KeyTextMessage"=w180, "RobotMessageArgument"=w179, "RobotMessageCode"=w178, "RobotMessageTitle"=w177) -> (w49:T8)  [unwired: 1 in]
  n60 = Bundle("BaudRate"=w75, "Parity"=w74, "RxIdleChars"=w73, "TxIdleChars"=w72, "ToolCommunicationIsEnabled"=w71, "StopBits"=w70) -> (w69:T9)  [unwired: 1 in]
  n61 = property class="JointData"(reference=w235) -> (reference out=w29:refnum<k24>, "ActualSpeed"=w234:dbl, "Current"=w233:sgl, "JointMode"=w232:u8, "Position"=w231:dbl, "TargetPosition"=w230:dbl, "Temperature"=w229:sgl, "Voltage"=w228:sgl)  [unwired: 1 in, 1 out]
  n62 = property class="JointData"(reference=w192) -> (reference out=w28:refnum<k24>, "ActualSpeed"=w221:dbl, "Current"=w222:sgl, "JointMode"=w223:u8, "Position"=w224:dbl, "TargetPosition"=w225:dbl, "Temperature"=w226:sgl, "Voltage"=w227:sgl)  [unwired: 1 in, 1 out]
  n63 = property class="JointData"(reference=w191) -> (reference out=w27:refnum<k24>, "ActualSpeed"=w220:dbl, "Current"=w219:sgl, "JointMode"=w218:u8, "Position"=w217:dbl, "TargetPosition"=w216:dbl, "Temperature"=w215:sgl, "Voltage"=w214:sgl)  [unwired: 1 in, 1 out]
  n64 = property class="JointData"(reference=w190) -> (reference out=w26:refnum<k24>, "ActualSpeed"=w193:dbl, "Current"=w194:sgl, "JointMode"=w195:u8, "Position"=w196:dbl, "TargetPosition"=w197:dbl, "Temperature"=w198:sgl, "Voltage"=w199:sgl)  [unwired: 1 in, 1 out]
  n65 = property class="JointData"(reference=w189) -> (reference out=w24:refnum<k24>, "ActualSpeed"=w206:dbl, "Current"=w205:sgl, "JointMode"=w204:u8, "Position"=w203:dbl, "TargetPosition"=w202:dbl, "Temperature"=w201:sgl, "Voltage"=w200:sgl)  [unwired: 1 in, 1 out]
  n66 = property class="JointData"(reference=w188) -> (reference out=w23:refnum<k24>, "ActualSpeed"=w207:dbl, "Current"=w208:sgl, "JointMode"=w209:u8, "Position"=w210:dbl, "TargetPosition"=w211:dbl, "Temperature"=w212:sgl, "Voltage"=w213:sgl)  [unwired: 1 in, 1 out]
  n67 = Close Reference(reference=w36) -> ()  [unwired: 1 in, 1 out]
  n68 = Close Reference(reference=w35) -> ()  [unwired: 1 in, 1 out]
  n69 = Close Reference(reference=w34) -> ()  [unwired: 1 in, 1 out]
  n70 = Close Reference(reference=w33) -> ()  [unwired: 1 in, 1 out]
  n71 = Close Reference(reference=w32) -> ()  [unwired: 1 in, 1 out]
  n72 = Close Reference(reference=w31) -> ()  [unwired: 1 in, 1 out]
  n73 = Close Reference(reference=w29) -> ()  [unwired: 1 in, 1 out]
  n74 = Close Reference(reference=w28) -> ()  [unwired: 1 in, 1 out]
  n75 = Close Reference(reference=w27) -> ()  [unwired: 1 in, 1 out]
  n76 = Close Reference(reference=w26) -> ()  [unwired: 1 in, 1 out]
  n77 = Close Reference(reference=w24) -> ()  [unwired: 1 in, 1 out]
  n78 = Close Reference(reference=w23) -> ()  [unwired: 1 in, 1 out]
  n79 = Close Reference(reference=w22) -> ()  [unwired: 1 in, 1 out]
  n80 = Close Reference(reference=w21) -> ()  [unwired: 1 in, 1 out]
  n81 = Close Reference(reference=w20) -> ()  [unwired: 1 in, 1 out]
  n82 = Close Reference(reference=w19) -> ()  [unwired: 1 in, 1 out]
  n83 = Close Reference(reference=w18) -> ()  [unwired: 1 in, 1 out]
  n84 = Close Reference(reference=w17) -> ()  [unwired: 1 in, 1 out]
  n85 = Close Reference(reference=w13) -> ()  [unwired: 1 in, 1 out]
  n86 = Close Reference(reference=w12) -> ()  [unwired: 1 in, 1 out]
  n87 = Close Reference(reference=w6) -> ()  [unwired: 1 in, 1 out]
  n88 = Bundle("DHa"=w389, "DHalpha"=w388, "DHd"=w387, "DHtheta"=w385, "JointMaxAcceleration"=w386, "JointMaxLimit"=w384, "JointMaxSpeed"=w383, "JointMinLimit"=w382) -> (w327:T10)  [unwired: 1 in]
  n89 = Bundle("DHa"=w342, "DHalpha"=w343, "DHd"=w344, "DHtheta"=w346, "JointMaxAcceleration"=w345, "JointMaxLimit"=w347, "JointMaxSpeed"=w348, "JointMinLimit"=w349) -> (w326:T10)  [unwired: 1 in]
  n90 = Bundle("DHa"=w357, "DHalpha"=w356, "DHd"=w355, "DHtheta"=w353, "JointMaxAcceleration"=w354, "JointMaxLimit"=w352, "JointMaxSpeed"=w351, "JointMinLimit"=w350) -> (w325:T10)  [unwired: 1 in]
  n91 = Bundle("DHa"=w374, "DHalpha"=w375, "DHd"=w376, "DHtheta"=w378, "JointMaxAcceleration"=w377, "JointMaxLimit"=w379, "JointMaxSpeed"=w380, "JointMinLimit"=w381) -> (w324:T10)  [unwired: 1 in]
  n92 = Bundle("DHa"=w373, "DHalpha"=w372, "DHd"=w371, "DHtheta"=w369, "JointMaxAcceleration"=w370, "JointMaxLimit"=w368, "JointMaxSpeed"=w367, "JointMinLimit"=w366) -> (w323:T10)  [unwired: 1 in]
  n93 = Bundle("DHa"=w358, "DHalpha"=w359, "DHd"=w360, "DHtheta"=w362, "JointMaxAcceleration"=w361, "JointMaxLimit"=w363, "JointMaxSpeed"=w364, "JointMinLimit"=w365) -> (w322:T10)  [unwired: 1 in]
  n94 = Bundle("ActualSpeed"=w234, "Current"=w233, "JointMode"=w232, "Position"=w231, "TargetPosition"=w230, "Temperature"=w229, "Voltage"=w228) -> (w187:T11)  [unwired: 1 in]
  n95 = Bundle("ActualSpeed"=w221, "Current"=w222, "JointMode"=w223, "Position"=w224, "TargetPosition"=w225, "Temperature"=w226, "Voltage"=w227) -> (w186:T11)  [unwired: 1 in]
  n96 = Bundle("ActualSpeed"=w220, "Current"=w219, "JointMode"=w218, "Position"=w217, "TargetPosition"=w216, "Temperature"=w215, "Voltage"=w214) -> (w185:T11)  [unwired: 1 in]
  n97 = Bundle("ActualSpeed"=w193, "Current"=w194, "JointMode"=w195, "Position"=w196, "TargetPosition"=w197, "Temperature"=w198, "Voltage"=w199) -> (w184:T11)  [unwired: 1 in]
  n98 = Bundle("ActualSpeed"=w206, "Current"=w205, "JointMode"=w204, "Position"=w203, "TargetPosition"=w202, "Temperature"=w201, "Voltage"=w200) -> (w183:T11)  [unwired: 1 in]
  n99 = Bundle("ActualSpeed"=w207, "Current"=w208, "JointMode"=w209, "Position"=w210, "TargetPosition"=w211, "Temperature"=w212, "Voltage"=w213) -> (w182:T11)  [unwired: 1 in]
  n100 = Bundle("Checksum"=w320, "DHa"=w319, "Dhalpha"=w318, "DHd"=w317, "DHtheta"=w316) -> (w285:T12)  [unwired: 1 in]
  n101 = Bundle("Checksum"=w311, "DHa"=w312, "Dhalpha"=w313, "DHd"=w314, "DHtheta"=w315) -> (w284:T12)  [unwired: 1 in]
  n102 = Bundle("Checksum"=w310, "DHa"=w309, "Dhalpha"=w308, "DHd"=w307, "DHtheta"=w306) -> (w283:T12)  [unwired: 1 in]
  n103 = Bundle("Checksum"=w301, "DHa"=w302, "Dhalpha"=w303, "DHd"=w304, "DHtheta"=w305) -> (w282:T12)  [unwired: 1 in]
  n104 = Bundle("Checksum"=w300, "DHa"=w299, "Dhalpha"=w298, "DHd"=w297, "DHtheta"=w296) -> (w281:T12)  [unwired: 1 in]
  n105 = Bundle("Checksum"=w291, "DHa"=w292, "Dhalpha"=w293, "DHd"=w294, "DHtheta"=w295) -> (w280:T12)  [unwired: 1 in]
  n106 = Bundle("Configurable0"=w174, "Configurable1"=w173, "Configurable2"=w172, "Configurable3"=w171, "Configurable4"=w170, "Configurable5"=w169, "Configurable6"=w168, "Configurable7"=w167, "Digital0"=w166, "Digital1"=w165, "Digital2"=w164, "Digital3"=w163, "Digital4"=w162, "Digital5"=w161, "Digital6"=w160, "Digital7"=w159, "ToolDigital0"=w158, "ToolDigital1"=w157, "Value"=w156) -> (w127:T13)  [unwired: 1 in]
  n107 = Bundle("Configurable0"=w137, "Configurable1"=w138, "Configurable2"=w139, "Configurable3"=w140, "Configurable4"=w141, "Configurable5"=w142, "Configurable6"=w143, "Configurable7"=w144, "Digital0"=w145, "Digital1"=w146, "Digital2"=w147, "Digital3"=w148, "Digital4"=w149, "Digital5"=w150, "Digital6"=w151, "Digital7"=w152, "ToolDigital0"=w153, "ToolDigital1"=w154, "Value"=w155) -> (w126:T13)  [unwired: 1 in]
  n108 = Bundle("ControlMode"=w102, "EmergencyStopped"=w101, "PhysicalRobotConnected"=w100, "ProgramPaused"=w99, "ProgramRunning"=w98, "ProtectiveStopped"=w97, "RealRobotEnabled"=w96, "RobotMode"=w95, "RobotPowerOn"=w94, "SpeedScaling"=w93, "TargetSpeedFraction"=w92, "TargetSpeedFractionLimit"=w91, "TotalMilliseconds"=w51) -> (w85:T14)  [unwired: 1 in]
  n109 = Bundle("FreedriveButtonEnabled"=w271, "FreedriveButtonPressed"=w270, "IOEnabledFreedrive"=w269) -> (w43:T15)  [unwired: 1 in]
  n110 = Bundle("AJointDefault"=w336, "AToolDefault"=w335, "ControllerBoxType"=w334, "EqRadius"=w333, "MasterboardVersion"=w332, "RobotSubType"=w331, "RobotType"=w330, "VJointDefault"=w329, "VToolDefault"=w328, w327, w326, w325, w324, w323, w322) -> (w46:T16)  [unwired: 1 in]
  n111 = Bundle(w187, w186, w185, w184, w183, w182) -> (w48:T17)  [unwired: 1 in]
  n112 = Bundle(w285, w284, w283, w282, w281, w280, "CalibrationStatus"=w279) -> (w42:T18)  [unwired: 1 in]
  n113 = Bundle("AnalogInput0"=w135, "AnalogInput1"=w134, "AnalogInputRange0"=w133, "AnalogInputRange1"=w132, "AnalogOutput0"=w131, "AnalogOutput1"=w130, "AnalogOutputDomain0"=w129, "AnalogOutputDomain1"=w128, w127, w126, "Euromap67Installed"=w125, "EuromapCurrent"=w124, "EuromapInputBits"=w123, "EuromapOutputBits"=w122, "EuromapVoltage"=w121, "InReducedMode"=w120, "MasterboardTemperature"=w119, "MasterIOCurrent"=w118, "OperationalModeSelectorInput"=w117, "RobotCurrent"=w116, "RobotVoltage48V"=w115, "Safetymode"=w114, "ThreePositionEnablingDeviceInput"=w113) -> (w112:T19)  [unwired: 1 in]
  n114 = Bundle("RuntimeExceptionTextMessage"=w90, "ScriptColumnNumber"=w89, "ScriptLineNumber"=w88) -> (w84:T20)  [unwired: 1 in]
  n115 = Bundle("SingularitySeverity"=w82, "SingularityType"=w81) -> (w80:T21)  [unwired: 1 in]
  n116 = Bundle("TextMessage"=w78) -> (w77:cluster{"TextMessage":string})  [unwired: 1 in]
  n117 = Bundle("DigitalOutputMode0"=w57, "DigitalOutputMode1"=w56, "OutputMode"=w55) -> (w53:T22)  [unwired: 1 in]
  n118 = Bundle(w43, w44, w45, w46, w47, w48, w49, w42, w112, w86, w85, w84, w80, w77, w69, w54, w53, w52) -> (→"Data":T23)  [unwired: 1 in]
